vi "MeasureDialog.vi"(8 "Error In":errorcluster, 11 "Measure Configuration In":T1[](array[typedef]) {"Count" min=1 step=1}) -> (0 "Error Out":errorcluster, 2 "Cancelled?":bool, 3 "Measure Configuration Out":T1[](array[typedef]) {"Count" min=1 step=1})   [LabVIEW 2012]
uses:
  MeasureConfiguration.ctl
  libs/LV-Utilities/LV-Utilities.lvlib
panel:
  in  "SMU B Current Auto Range?":bool=TRUE
  in  "SMU B Low Limit Current (A)":dbl format="%_4p"
  in  "SMU B High Limit Current (A)":dbl format="%_4p"
  in  "SMU B Voltage Auto Range?":bool=TRUE
  in  "SMU B Low Limit Voltage (V)":dbl format="%_4p"
  in  "SMU B High Limit Voltage (V)":dbl format="%_4p"
  in  "SMU B Active?":bool=TRUE
  in  "SMU B Interval (sec)":dbl=0.01 format="%_4p"
  in  "SMU B Count":u8=1 min=1 step=1
  in  "SMU A Active?":bool=TRUE
  in  "SMU A Interval (sec)":dbl=0.01 format="%_4p"
  in  "SMU A Count":u8=1 min=1 step=1
  in  "SMU A Current Auto Range?":bool=TRUE
  in  "SMU A Low Limit Current (A)":dbl format="%_4p"
  in  "SMU A High Limit Current (A)":dbl format="%_4p"
  in  "SMU A Voltage Auto Range?":bool=TRUE
  in  "SMU A Low Limit Voltage (V)":dbl format="%_4p"
  in  "SMU A High Limit Voltage (V)":dbl format="%_4p"
  in  "CANCEL":bool
  in  "DONE":bool
  # "SOURCE-MEASURE UNIT B"
  # "Current Range"
  # "Auto"
  # "Low Limit"
  # "High Limit"
  # "Voltage Range"
  # "Auto"
  # "Low Limit"
  # "High Limit"
  # "General"
  # "Active"
  # "Interval"
  # "Count"
  # "SOURCE-MEASURE UNIT A"
  # "General"
  # "Active"
  # "Interval"
  # "Count"
  # "Current Range"
  # "Auto"
  # "Low Limit"
  # "High Limit"
  # "Voltage Range"
  # "Auto"
  # "Low Limit"
  # "High Limit"
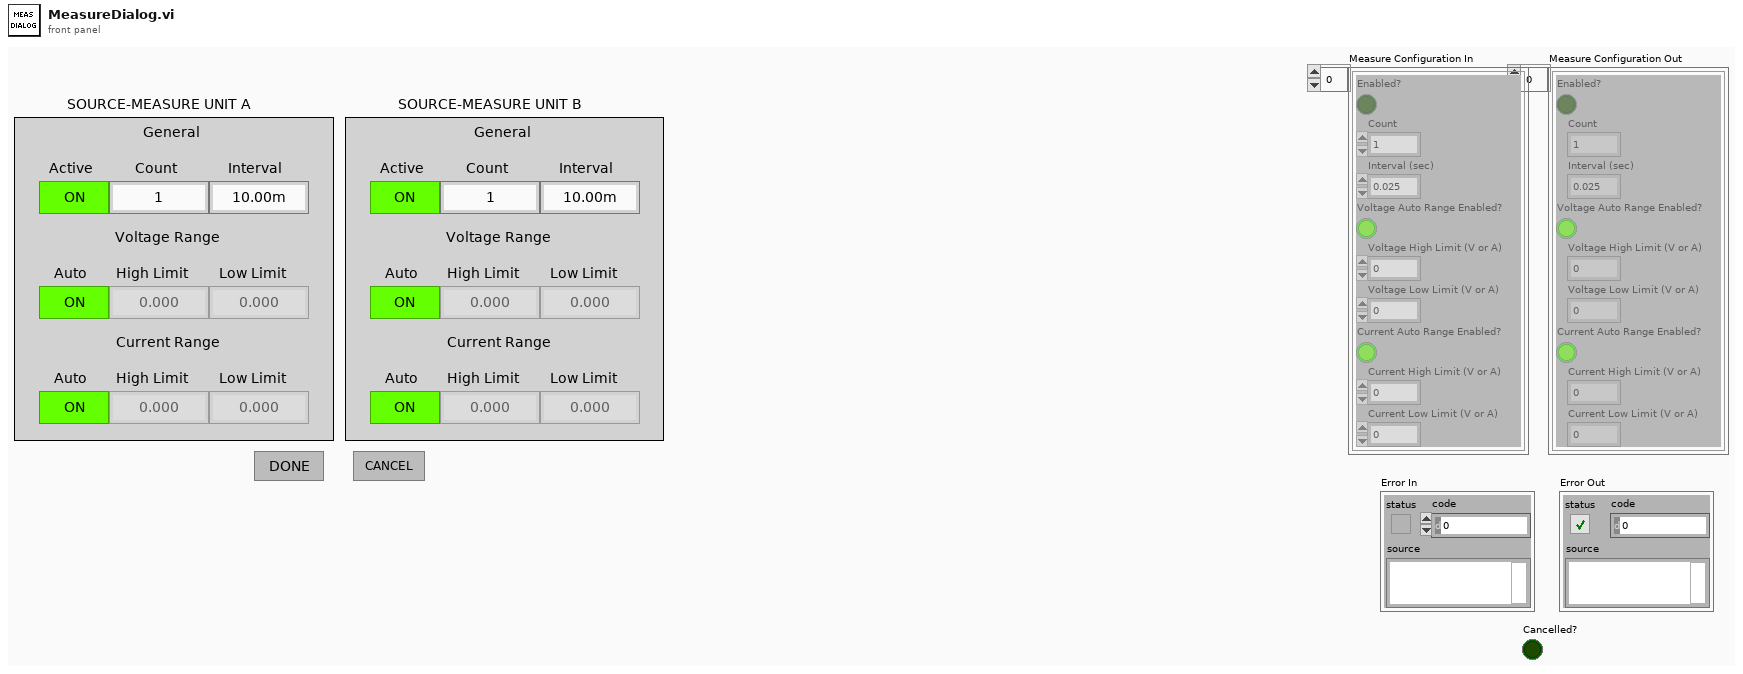
[diagram p1: front panel]
types:
  T1 = typedef "MeasureConfiguration.ctl" = cluster{"Enabled?":bool, "Count":u8, "Interval (sec)":dbl, "Voltage Auto Range Enabled?":bool, "Voltage High Limit (V or A)":dbl, "Voltage Low Limit (V or A)":dbl, "Current Auto Range Enabled?":bool, "Current High Limit (V or A)":dbl, "Current Low Limit (V or A)":dbl}
  T2 = enum8{"Enabled", "Disabled", "Disabled and Grayed Out"}
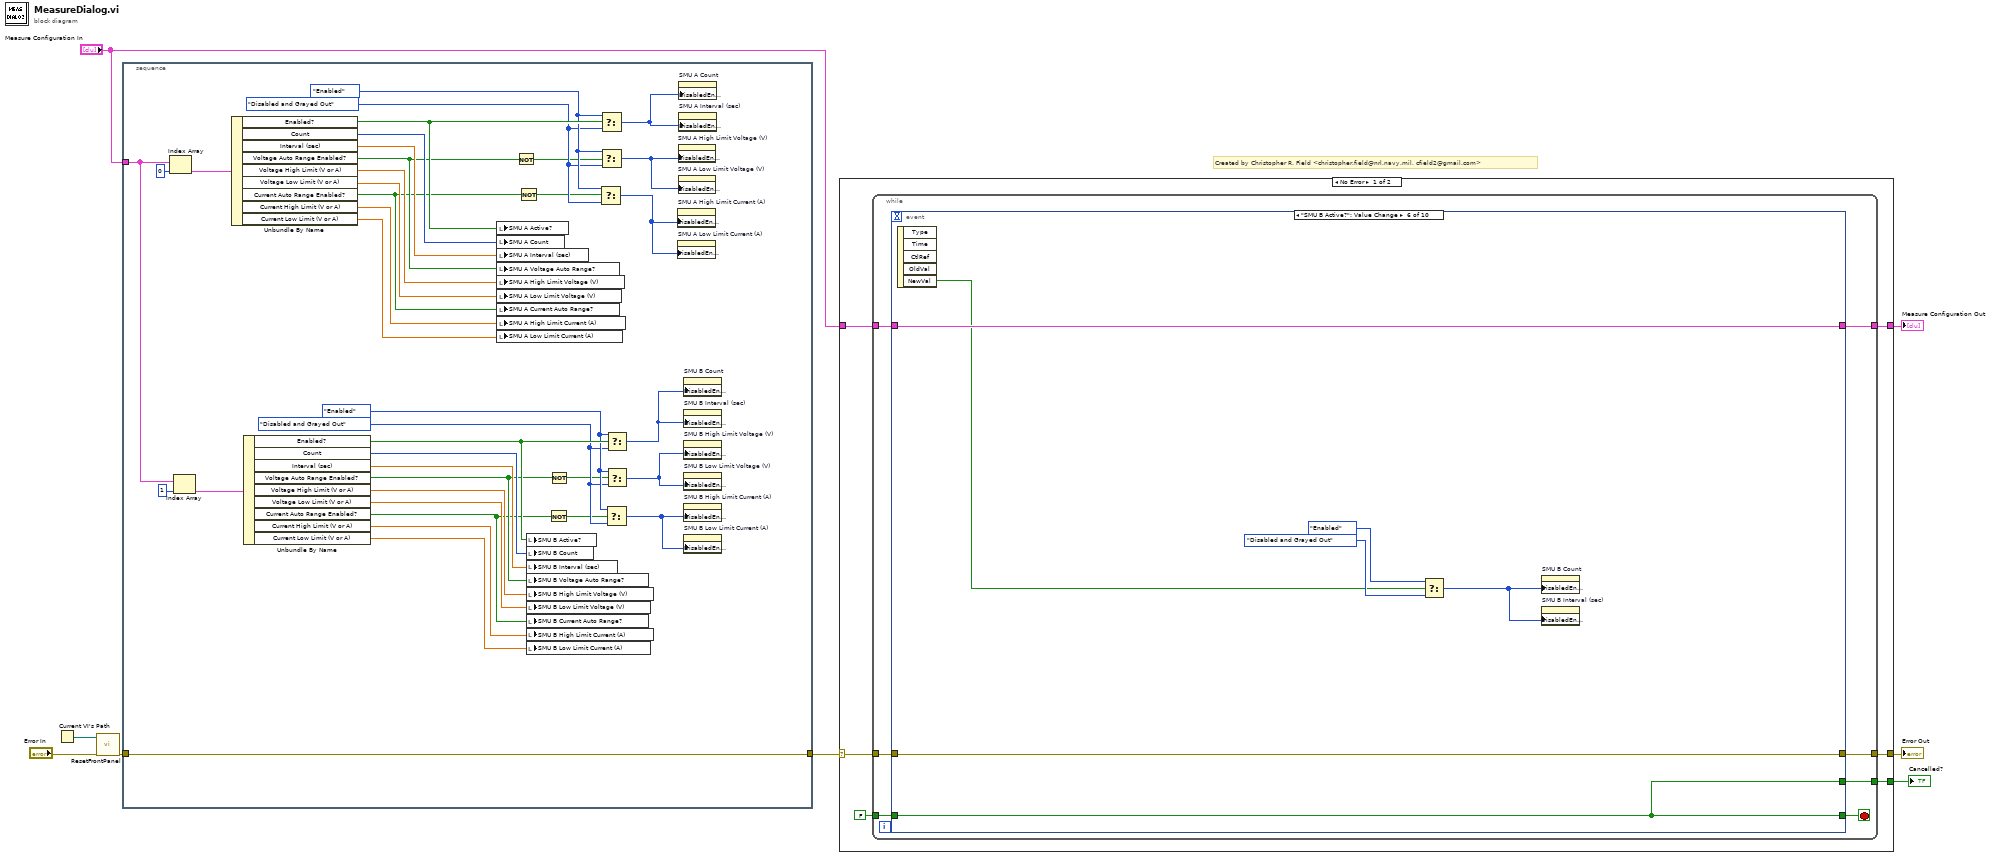
[diagram p0: block diagram]
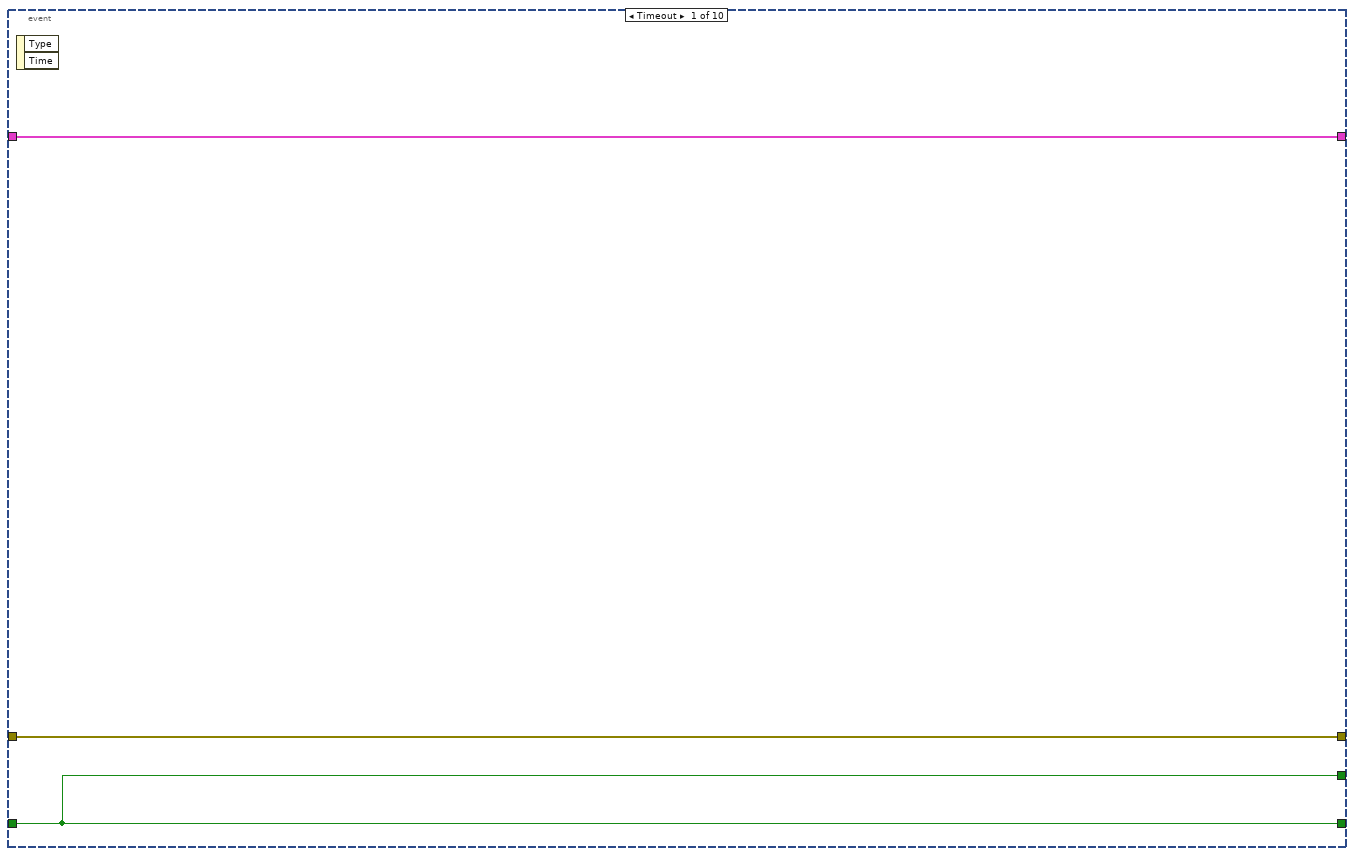
[diagram p2: hidden frame]
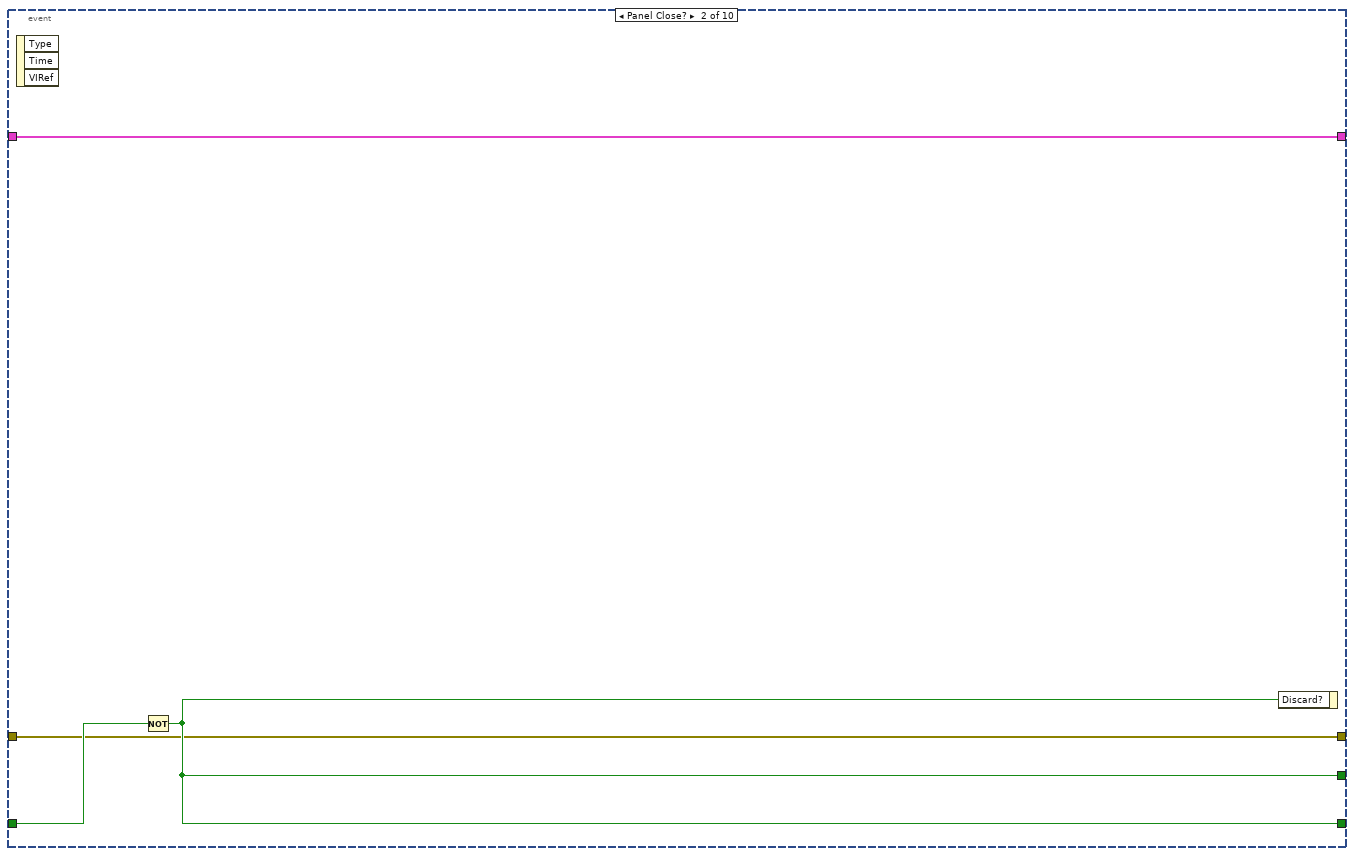
[diagram p3: hidden frame]
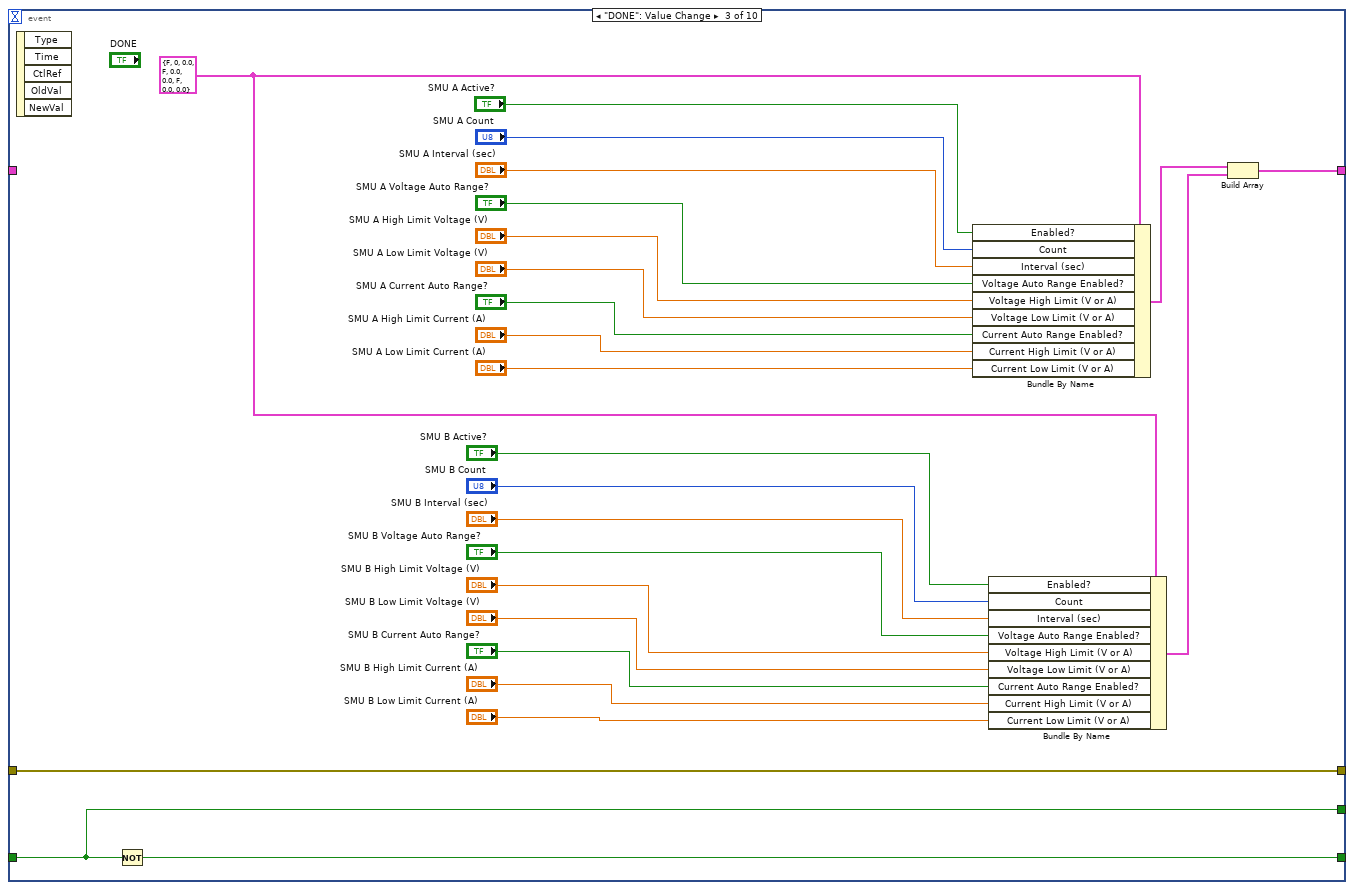
[diagram p4: hidden frame]
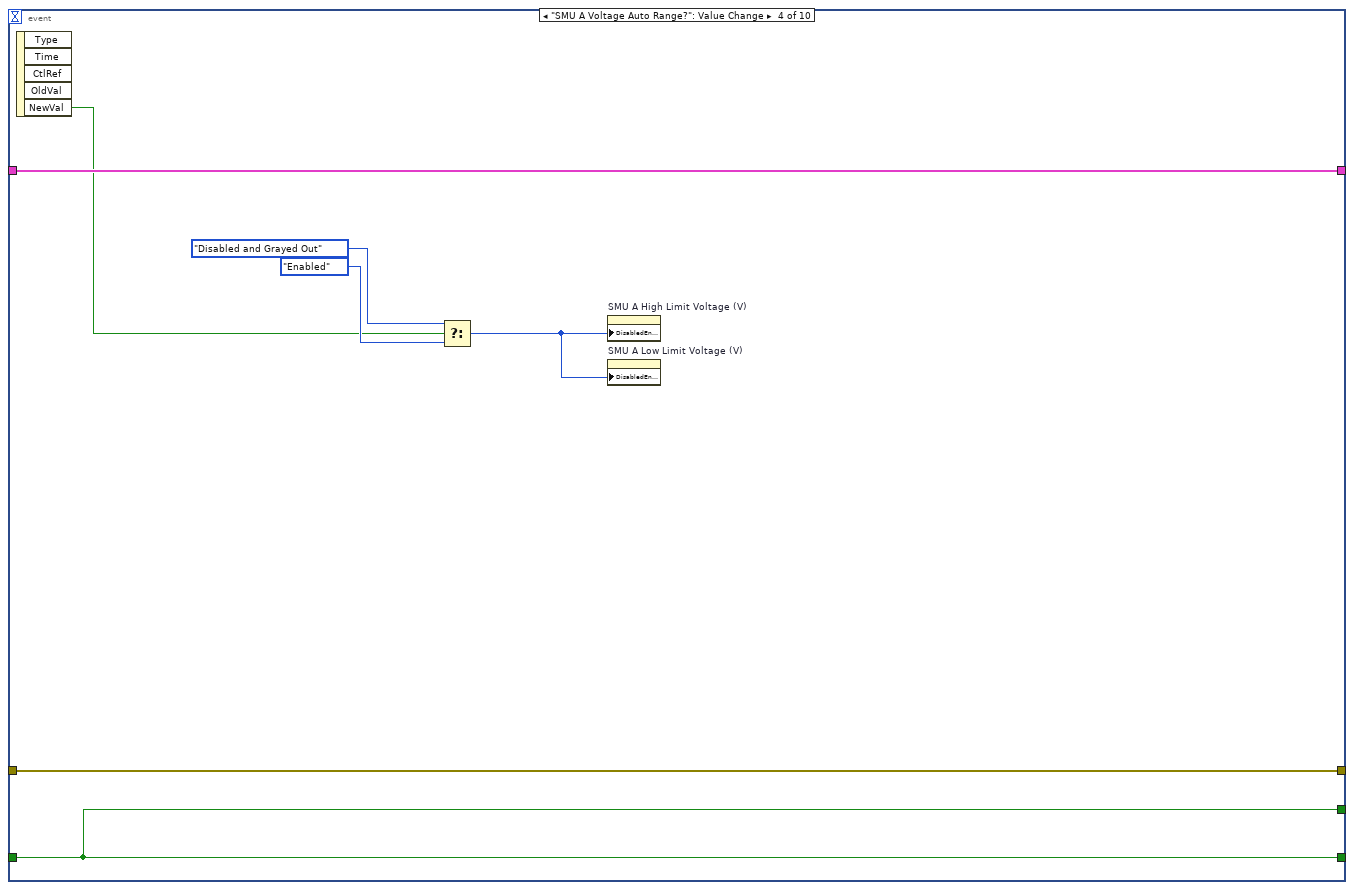
[diagram p5: hidden frame]
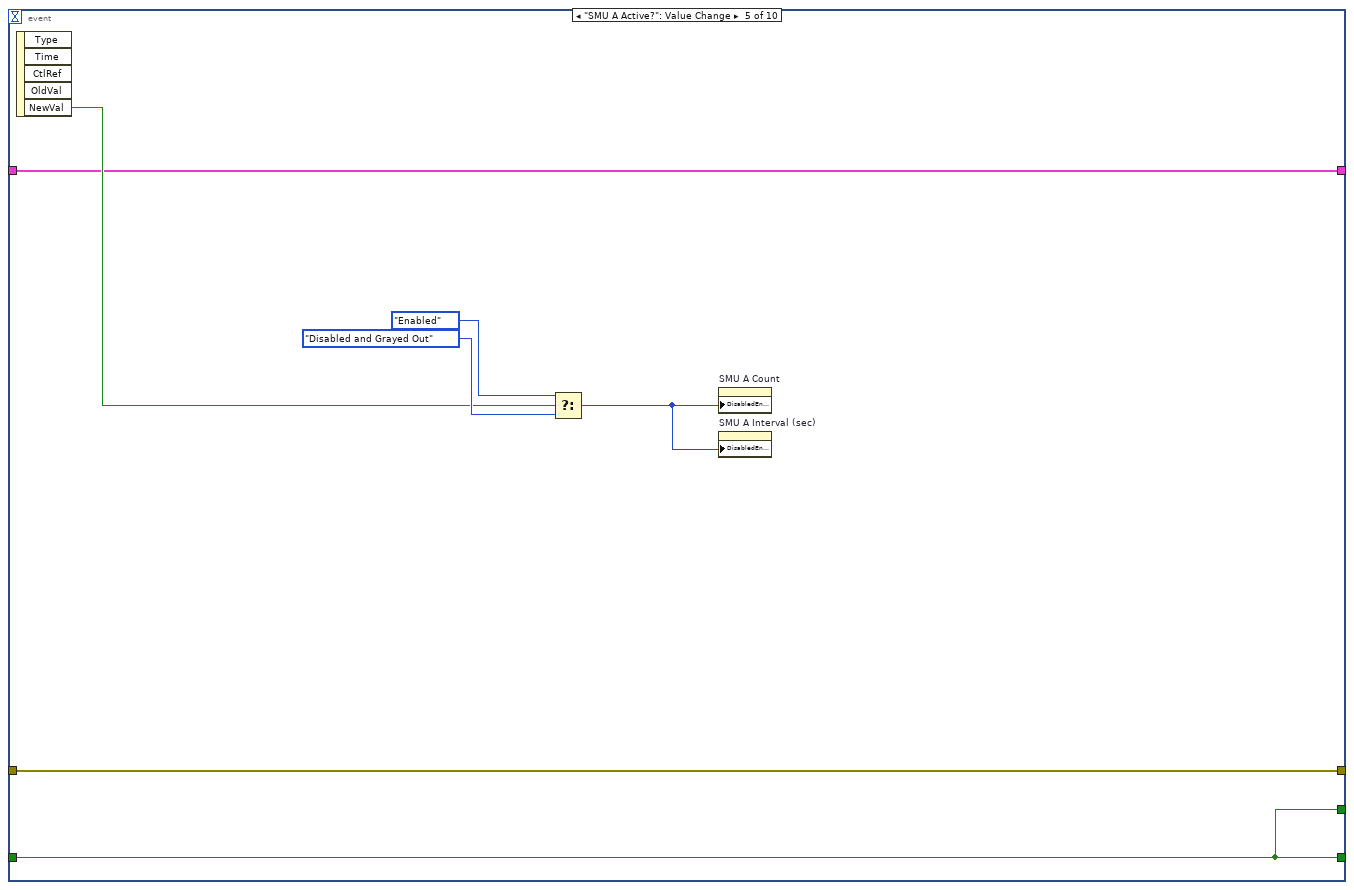
[diagram p6: hidden frame]
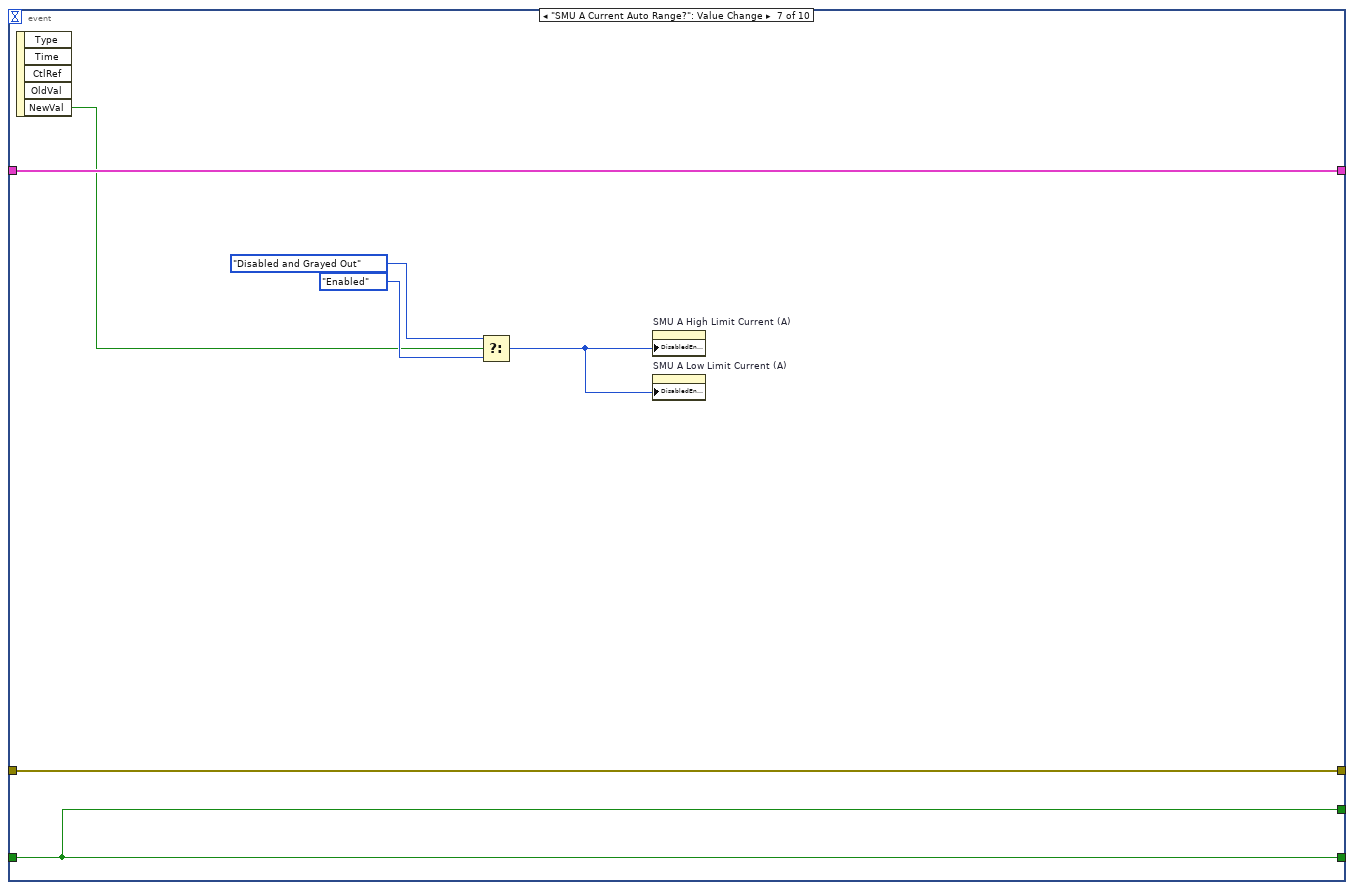
[diagram p7: hidden frame]
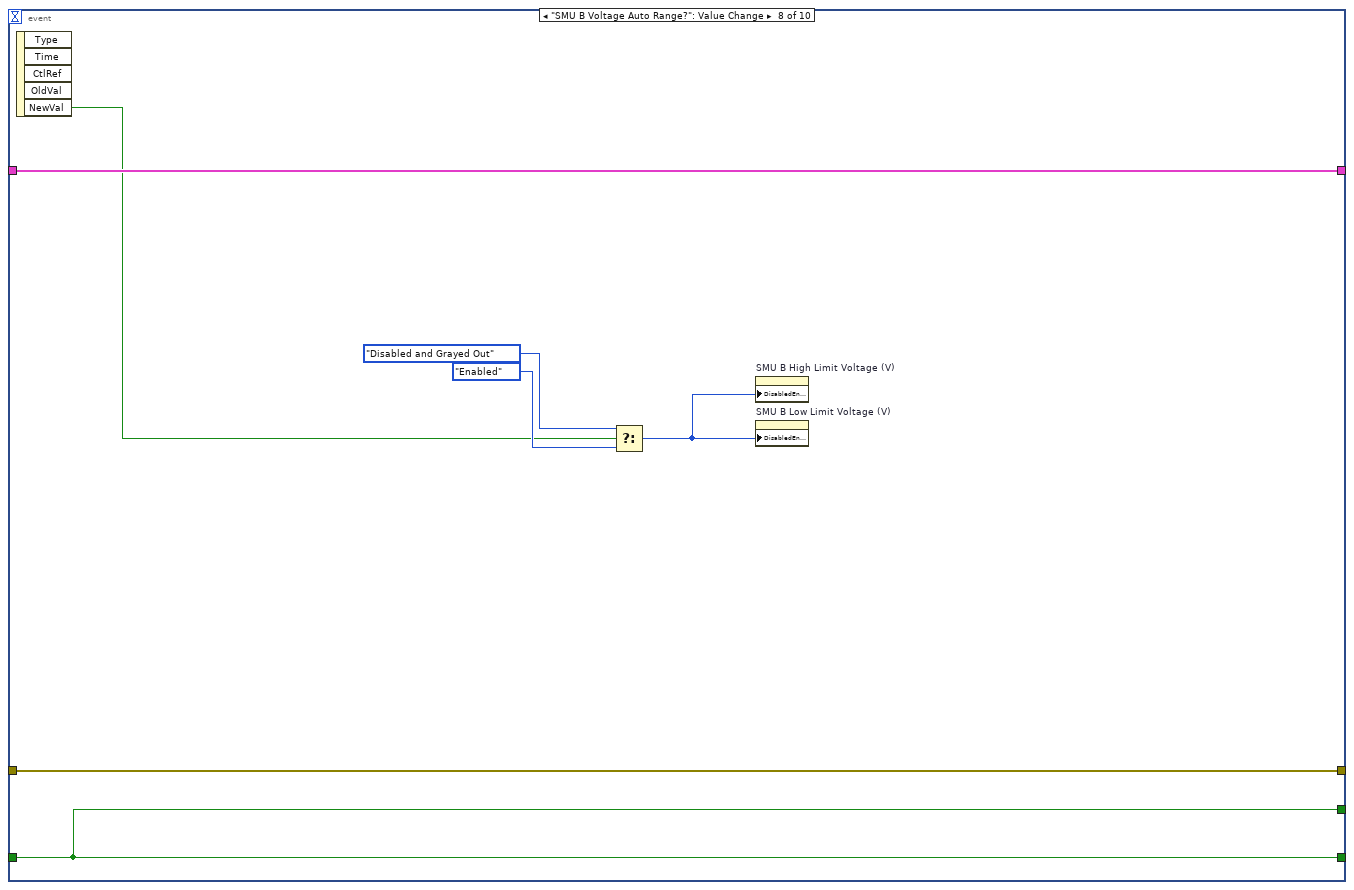
[diagram p8: hidden frame]
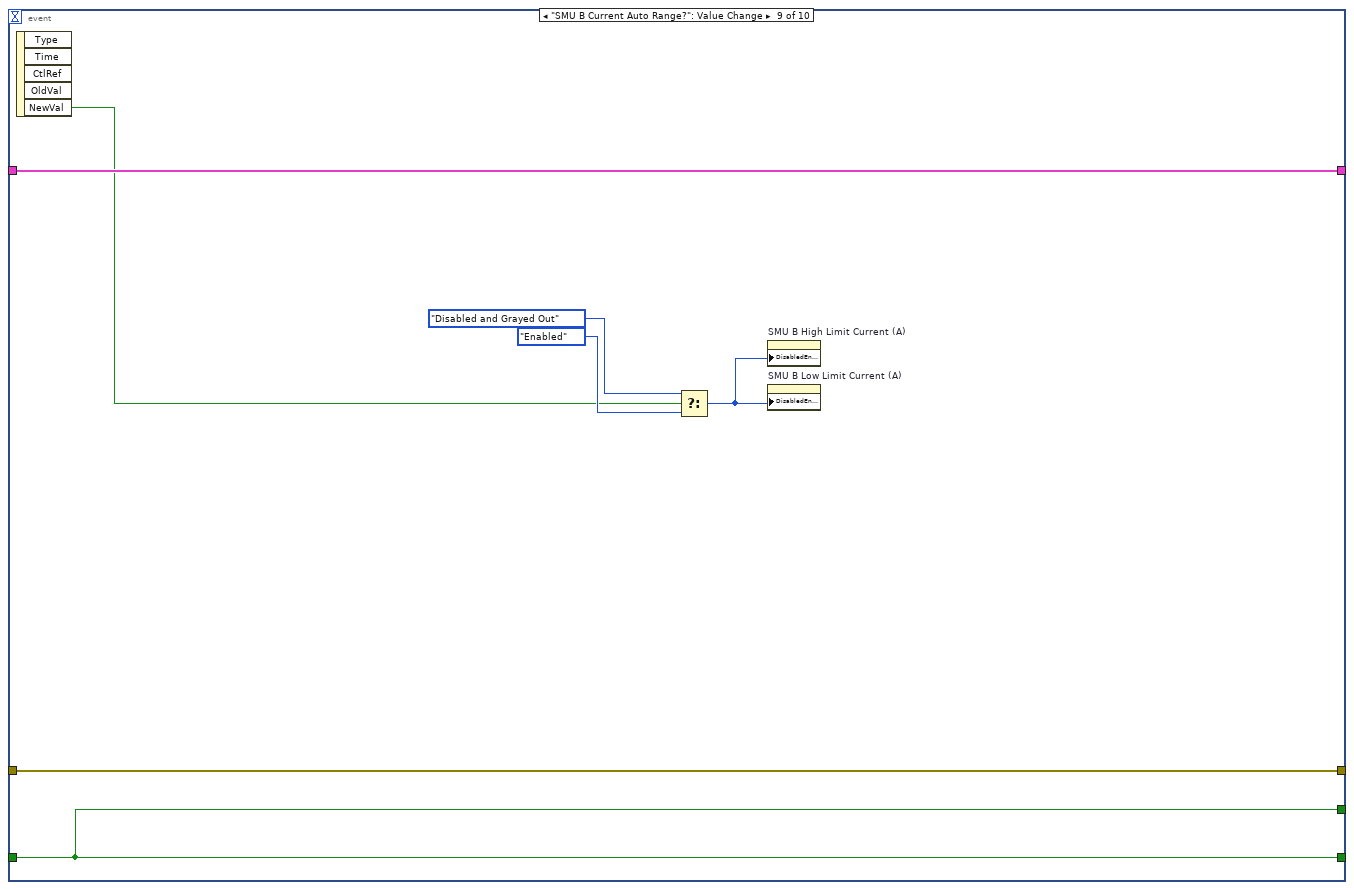
[diagram p9: hidden frame]
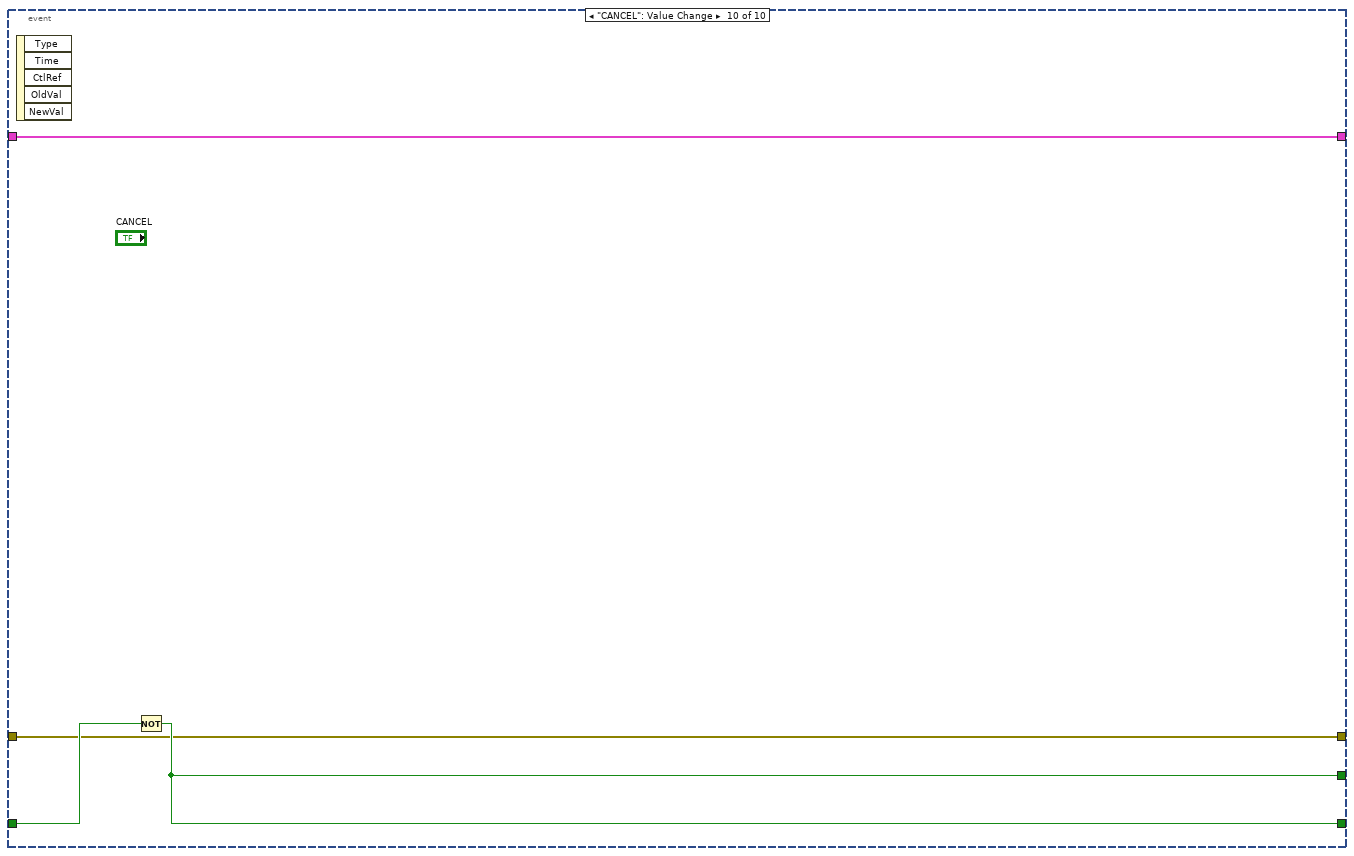
[diagram p10: hidden frame]
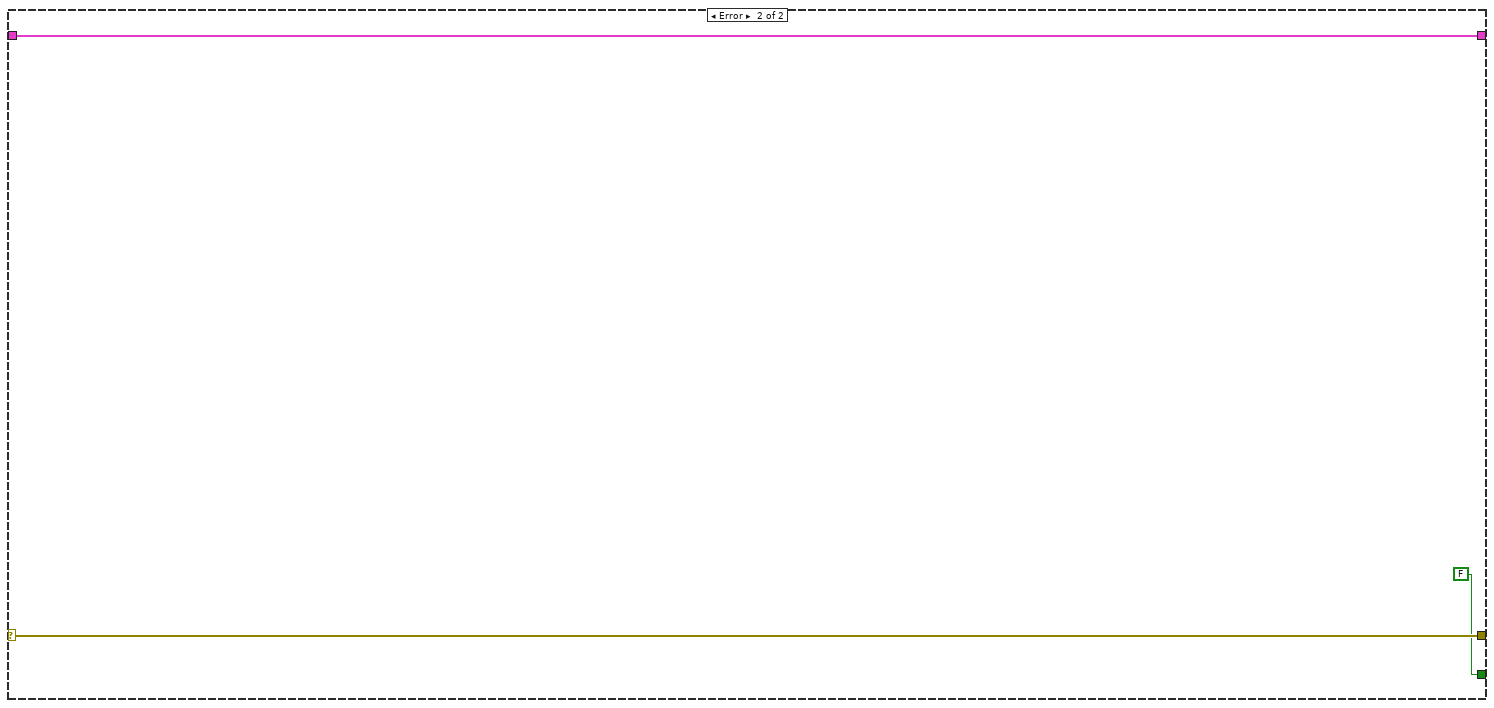
[diagram p11: hidden frame]
diagram:
  # "Created by Christopher R. Field <christopher.field@nrl.navy.mil, cfield2@gmail.com>"
  n1 = Current VI's Path() -> (path=w7:path)
  n2 = call "ResetFrontPanel.vi"("Error In"="Error In", "VI Path"=w7) -> ("Error Out"=w5:errorcluster)  [unwired: 9 in]
  n3 = stacked-sequence {
    tunnel: w5 -> [w46]
    tunnel: [w46] -> w4
    tunnel: "Measure Configuration In" -> [w37]
    frame #0 {
      w20 = T2."Disabled and Grayed Out" ("Disabled")
      w21 = T2."Enabled" ("Disabled")
      w24 = T2."Disabled and Grayed Out" ("Disabled")
      w25 = T2."Enabled" ("Disabled")
      n4 = Index Array(array=w37, index=0) -> (element=w44:T1)
      n5 = Index Array(array=w37, index=1) -> (element=w42:T1)
      n6 = Unbundle By Name(w44) -> ("Enabled?"=w26:bool, "Count"=w34:u8, "Interval (sec)"=w33:dbl, "Voltage Auto Range Enabled?"=w12:bool, "Voltage High Limit (V or A)"=w32:dbl, "Voltage Low Limit (V or A)"=w31:dbl, "Current Auto Range Enabled?"=w10:bool, "Current High Limit (V or A)"=w30:dbl, "Current Low Limit (V or A)"=w29:dbl)
      n7 = Unbundle By Name(w42) -> ("Enabled?"=w22:bool, "Count"=w41:u8, "Interval (sec)"=w40:dbl, "Voltage Auto Range Enabled?"=w16:bool, "Voltage High Limit (V or A)"=w39:dbl, "Voltage Low Limit (V or A)"=w38:dbl, "Current Auto Range Enabled?"=w14:bool, "Current High Limit (V or A)"=w36:dbl, "Current Low Limit (V or A)"=w35:dbl)
      n8 = local write "SMU A Active?"(w26) -> ()
      n9 = local write "SMU A Count"(w34) -> ()
      n10 = local write "SMU A Interval (sec)"(w33) -> ()
      n11 = local write "SMU A Voltage Auto Range?"(w12) -> ()
      n12 = local write "SMU A High Limit Voltage (V)"(w32) -> ()
      n13 = local write "SMU A Low Limit Voltage (V)"(w31) -> ()
      n14 = local write "SMU A Current Auto Range?"(w10) -> ()
      n15 = local write "SMU A High Limit Current (A)"(w30) -> ()
      n16 = local write "SMU A Low Limit Current (A)"(w29) -> ()
      n17 = Not(x=w12) -> (.not. x?=w11:bool)
      n18 = Not(x=w10) -> (.not. x?=w9:bool)
      n19 = local write "SMU B Active?"(w22) -> ()
      n20 = local write "SMU B Count"(w41) -> ()
      n21 = local write "SMU B Interval (sec)"(w40) -> ()
      n22 = local write "SMU B Voltage Auto Range?"(w16) -> ()
      n23 = local write "SMU B High Limit Voltage (V)"(w39) -> ()
      n24 = local write "SMU B Low Limit Voltage (V)"(w38) -> ()
      n25 = local write "SMU B Current Auto Range?"(w14) -> ()
      n26 = local write "SMU B High Limit Current (A)"(w36) -> ()
      n27 = local write "SMU B Low Limit Current (A)"(w35) -> ()
      n28 = Not(x=w14) -> (.not. x?=w13:bool)
      n29 = Not(x=w16) -> (.not. x?=w15:bool)
      n30 = Select(t=w25, s=w9, f=w24) -> (s? t:f=w27:T2)
      n31 = Select(t=w25, s=w26, f=w24) -> (s? t:f=w23:T2)
      n32 = Select(t=w25, s=w11, f=w24) -> (s? t:f=w28:T2)
      n33 = Select(t=w21, s=w13, f=w20) -> (s? t:f=w18:T2)
      n34 = Select(t=w21, s=w22, f=w20) -> (s? t:f=w17:T2)
      n35 = Select(t=w21, s=w15, f=w20) -> (s? t:f=w19:T2)
      n36 = property on="SMU A High Limit Current (A)" class="DigNum (strict)"("DisabledEnum"=w27) -> ()  [unwired: 2 in, 2 out]
      n37 = property on="SMU A Low Limit Current (A)" class="DigNum (strict)"("DisabledEnum"=w27) -> ()  [unwired: 2 in, 2 out]
      n38 = property on="SMU A High Limit Voltage (V)" class="DigNum (strict)"("DisabledEnum"=w28) -> ()  [unwired: 2 in, 2 out]
      n39 = property on="SMU A Low Limit Voltage (V)" class="DigNum (strict)"("DisabledEnum"=w28) -> ()  [unwired: 2 in, 2 out]
      n40 = property on="SMU A Count" class="DigNum (strict)"("DisabledEnum"=w23) -> ()  [unwired: 2 in, 2 out]
      n41 = property on="SMU A Interval (sec)" class="DigNum (strict)"("DisabledEnum"=w23) -> ()  [unwired: 2 in, 2 out]
      n42 = property on="SMU B Count" class="DigNum (strict)"("DisabledEnum"=w17) -> ()  [unwired: 2 in, 2 out]
      n43 = property on="SMU B Interval (sec)" class="DigNum (strict)"("DisabledEnum"=w17) -> ()  [unwired: 2 in, 2 out]
      n44 = property on="SMU B High Limit Voltage (V)" class="DigNum (strict)"("DisabledEnum"=w19) -> ()  [unwired: 2 in, 2 out]
      n45 = property on="SMU B Low Limit Voltage (V)" class="DigNum (strict)"("DisabledEnum"=w19) -> ()  [unwired: 2 in, 2 out]
      n46 = property on="SMU B High Limit Current (A)" class="DigNum (strict)"("DisabledEnum"=w18) -> ()  [unwired: 2 in, 2 out]
      n47 = property on="SMU B Low Limit Current (A)" class="DigNum (strict)"("DisabledEnum"=w18) -> ()  [unwired: 2 in, 2 out]
    }
  }
  n48 = case shown="No Error" w4 {
    selector: w4 -> [w50 w140]
    tunnel: [w51 FALSE] -> w8
    tunnel: [w49 w140] -> w3
    tunnel: [w48 w138] -> w2
    tunnel: "Measure Configuration In" -> [w47 w138]
    frame No Error {
      n49 = while {
        tunnel: FALSE -> [w59]
        tunnel: [w57] -> w51
        tunnel: w50 -> [w56]
        tunnel: [w55] -> w49
        tunnel: [w54] -> w48
        tunnel: w47 -> [w53]
        stop <- w58 stop-if-true
        n50 = event shown="[5] \"SMU B Active?\": Value Change" {
          selector: _ -> [_ _ _ _ _ _ _ _ _ _]
          dyn-events: _ -> [_ _ _ _ _ _ _ _ _ _]
          timeout: _ -> [_ _ _ _ _ _ _ _ _ _]
          tunnel: w59 -> [w62 w66 w90 w97 w99 w106 w117 w124 w131 w137]
          tunnel: [w62 w65 w91 w97 w99 w106 w117 w124 w131 w136] -> w58
          tunnel: [w62 w65 w90 w97 w99 w106 w117 w124 w131 w136] -> w57
          tunnel: w56 -> [w61 w64 w89 w98 w100 w107 w118 w125 w132 w135]
          tunnel: [w61 w64 w89 w98 w100 w107 w118 w125 w132 w135] -> w55
          tunnel: [w60 w63 w77 w96 w101 w109 w119 w126 w133 w134] -> w54
          tunnel: w53 -> [w60 w63 _ w96 w101 w109 w119 w126 w133 w134]
          event Timeout {
            n51 = event-data() -> ()  [unwired: 1 in, 2 out]
          }
          event Panel Close? {
            n52 = event-data() -> ()  [unwired: 1 in, 3 out]
            n53 = Not(x=w66) -> (.not. x?=w65:bool)
            n54 = event-data("Discard?"=w65) -> ()  [unwired: 1 in, 1 out]
          }
          event "DONE": Value Change {
            w84 = T1 {"Enabled?"=FALSE, "Count"=0, "Interval (sec)"=0.0, "Voltage Auto Range Enabled?"=FALSE, "Voltage High Limit (V or A)"=0.0, "Voltage Low Limit (V or A)"=0.0, "Current Auto Range Enabled?"=FALSE, "Current High Limit (V or A)"=0.0, "Current Low Limit (V or A)"=0.0} ("Measure Configuration")
            n55 = event-data() -> ()  [unwired: 1 in, 5 out]
            n56 = Not(x=w90) -> (.not. x?=w91:bool)
            n57 = Bundle By Name(cluster=w84, "Enabled?"="SMU A Active?", "Count"="SMU A Count", "Interval (sec)"="SMU A Interval (sec)", "Voltage Auto Range Enabled?"="SMU A Voltage Auto Range?", "Voltage High Limit (V or A)"="SMU A High Limit Voltage (V)", "Voltage Low Limit (V or A)"="SMU A Low Limit Voltage (V)", "Current Auto Range Enabled?"="SMU A Current Auto Range?", "Current High Limit (V or A)"="SMU A High Limit Current (A)", "Current Low Limit (V or A)"="SMU A Low Limit Current (A)") -> (w79:T1)
            n58 = Bundle By Name(cluster=w84, "Enabled?"="SMU B Active?", "Count"="SMU B Count", "Interval (sec)"="SMU B Interval (sec)", "Voltage Auto Range Enabled?"="SMU B Voltage Auto Range?", "Voltage High Limit (V or A)"="SMU B High Limit Voltage (V)", "Voltage Low Limit (V or A)"="SMU B Low Limit Voltage (V)", "Current Auto Range Enabled?"="SMU B Current Auto Range?", "Current High Limit (V or A)"="SMU B High Limit Current (A)", "Current Low Limit (V or A)"="SMU B Low Limit Current (A)") -> (w78:T1)
            n59 = Build Array(w79, w78) -> (w77:T1[])
          }
          event "SMU A Voltage Auto Range?": Value Change {
            n60 = event-data() -> ("NewVal"=w93:bool)  [unwired: 1 in, 4 out]
            n61 = Select(t=T2."Disabled and Grayed Out" ("Disabled"), s=w93, f=T2."Enabled" ("Disabled")) -> (s? t:f=w92:T2)
            n62 = property on="SMU A High Limit Voltage (V)" class="DigNum (strict)"("DisabledEnum"=w92) -> ()  [unwired: 2 in, 2 out]
            n63 = property on="SMU A Low Limit Voltage (V)" class="DigNum (strict)"("DisabledEnum"=w92) -> ()  [unwired: 2 in, 2 out]
          }
          event "SMU A Active?": Value Change {
            n64 = event-data() -> ("NewVal"=w102:bool)  [unwired: 1 in, 4 out]
            n65 = Select(t=T2."Enabled" ("Disabled"), s=w102, f=T2."Disabled and Grayed Out" ("Disabled")) -> (s? t:f=w103:T2)
            n66 = property on="SMU A Count" class="DigNum (strict)"("DisabledEnum"=w103) -> ()  [unwired: 2 in, 2 out]
            n67 = property on="SMU A Interval (sec)" class="DigNum (strict)"("DisabledEnum"=w103) -> ()  [unwired: 2 in, 2 out]
          }
          event "SMU B Active?": Value Change {
            n68 = event-data() -> ("NewVal"=w108:bool)  [unwired: 1 in, 4 out]
            n69 = Select(t=T2."Enabled" ("Disabled"), s=w108, f=T2."Disabled and Grayed Out" ("Disabled")) -> (s? t:f=w110:T2)
            n70 = property on="SMU B Count" class="DigNum (strict)"("DisabledEnum"=w110) -> ()  [unwired: 2 in, 2 out]
            n71 = property on="SMU B Interval (sec)" class="DigNum (strict)"("DisabledEnum"=w110) -> ()  [unwired: 2 in, 2 out]
          }
          event "SMU A Current Auto Range?": Value Change {
            n72 = event-data() -> ("NewVal"=w114:bool)  [unwired: 1 in, 4 out]
            n73 = Select(t=T2."Disabled and Grayed Out" ("Disabled"), s=w114, f=T2."Enabled" ("Disabled")) -> (s? t:f=w113:T2)
            n74 = property on="SMU A High Limit Current (A)" class="DigNum (strict)"("DisabledEnum"=w113) -> ()  [unwired: 2 in, 2 out]
            n75 = property on="SMU A Low Limit Current (A)" class="DigNum (strict)"("DisabledEnum"=w113) -> ()  [unwired: 2 in, 2 out]
          }
          event "SMU B Voltage Auto Range?": Value Change {
            n76 = event-data() -> ("NewVal"=w121:bool)  [unwired: 1 in, 4 out]
            n77 = Select(t=T2."Disabled and Grayed Out" ("Disabled"), s=w121, f=T2."Enabled" ("Disabled")) -> (s? t:f=w120:T2)
            n78 = property on="SMU B High Limit Voltage (V)" class="DigNum (strict)"("DisabledEnum"=w120) -> ()  [unwired: 2 in, 2 out]
            n79 = property on="SMU B Low Limit Voltage (V)" class="DigNum (strict)"("DisabledEnum"=w120) -> ()  [unwired: 2 in, 2 out]
          }
          event "SMU B Current Auto Range?": Value Change {
            n80 = event-data() -> ("NewVal"=w128:bool)  [unwired: 1 in, 4 out]
            n81 = Select(t=T2."Disabled and Grayed Out" ("Disabled"), s=w128, f=T2."Enabled" ("Disabled")) -> (s? t:f=w127:T2)
            n82 = property on="SMU B High Limit Current (A)" class="DigNum (strict)"("DisabledEnum"=w127) -> ()  [unwired: 2 in, 2 out]
            n83 = property on="SMU B Low Limit Current (A)" class="DigNum (strict)"("DisabledEnum"=w127) -> ()  [unwired: 2 in, 2 out]
          }
          event "CANCEL": Value Change {
            n84 = event-data() -> ()  [unwired: 1 in, 5 out]
            n85 = Not(x=w137) -> (.not. x?=w136:bool)
          }
        }
      }
    }
    frame Error {
    }
  }
  "Cancelled?" <- w8
  "Error Out" <- w3
  "Measure Configuration Out" <- w2
